vi "GT Set Gear Event.vi"(6 "startPara1":i32, 7 "startPara0":i32, 8 "error in (no error)":errorcluster caption="错误输入（无错误）", 9 "event":i16, 10 "profile":i16, 11 "cardNum":i16) -> (0 "error out":errorcluster caption="错误输出", 3 "function return":i16)   [LabVIEW 2014, in "gts.lvlib"]
doc: "GT_API GT_SetGearEvent(short cardNum,short profile,short event,long startPara0,long startPara1);"
uses:
  gts.lvlib
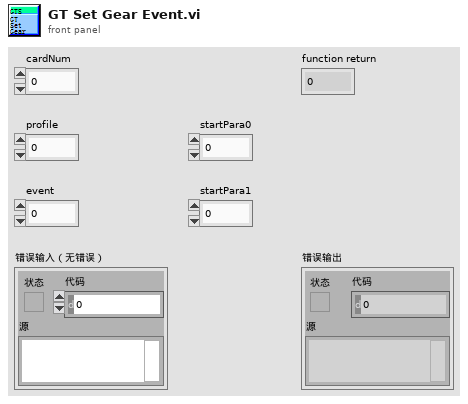
[diagram p1: front panel]
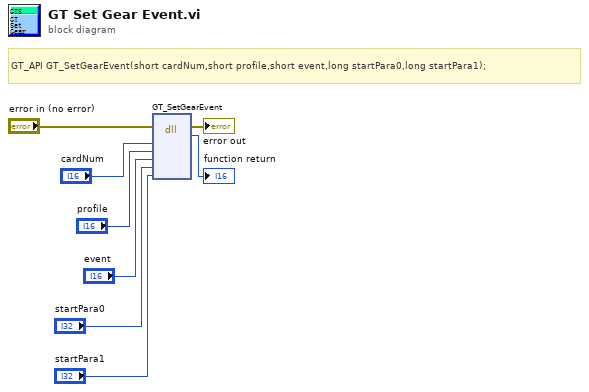
[diagram p0: block diagram]
diagram:
  # "GT_API GT_SetGearEvent(short cardNum,short profile,short event,long startPara0,long startPara1);"
  n1 = dll-call lib="PTH2habs D固高科技资料GTS控制卡GTS卡18年上半年资料dllVC32bit\nmulti_cardgts.*" fn="GT_SetGearEvent"(error in="error in (no error)", "cardNum"="cardNum", "profile"="profile", "event"="event", "startPara0"="startPara0", "startPara1"="startPara1") -> (error out=→"error out":errorcluster, →"function return":i16)  [unwired: 7 in, 1 out]
